vi "Get Pre and Post Build Actions.vi"(8 "error in (no error)":errorcluster, 11 "Build in":refnum<class "NI_AB_API_SDIST.lvclass">) -> (0 "error out":errorcluster, 1 "Post Build Action VI":refnum<vi>, 2 "Pre Build Action VI":refnum<vi>, 3 "Build out":refnum<class "NI_AB_API_SDIST.lvclass">)   [LabVIEW 2020, in "NI_AB_API_SDIST.lvclass"]
uses:
  <vilib>/AppBuilder/AB_API/SDIST/NI_AB_API_SDIST.lvclass
  <vilib>/AppBuilder/AB_API/SDIST/NI_AB_API_SDIST.lvclass/NI_AB_API_SDIST.ctl
  <vilib>/AppBuilder/AB_API/Build/NI_AB_API_Build.lvclass
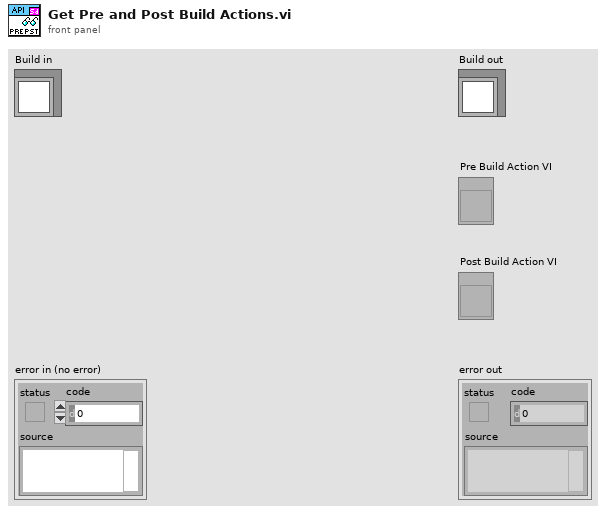
[diagram p1: front panel]
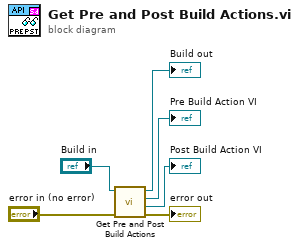
[diagram p0: block diagram]
diagram:
  n1 = call-parent "Get Pre and Post Build Actions.vi"("error in (no error)"="error in (no error)", "Build in"="Build in") -> ("error out"=→"error out":errorcluster, "Post Build Action VI"=→"Post Build Action VI":refnum<vi>, "Pre Build Action VI"=→"Pre Build Action VI":refnum<vi>, "Build out"=→"Build out":refnum<class "NI_AB_API_SDIST.lvclass">)  [unwired: 6 in]
